vi "Read Scaled Async Data.vi"(8 "error in (no error)":errorcluster, 10 "Async Message":refnum<class "Async Message.lvclass">, 11 "1553 Component in":refnum<class "1553 Component.lvclass">) -> (0 "error out":errorcluster, 1 "Scaled Data":dbl[](array[numeric]), 2 "Parameters":string[](array[string]), 3 "1553 Component out":refnum<class "1553 Component.lvclass">)   [LabVIEW 2020, in "BCI-1553 API.lvlib" / "1553 Component.lvclass"]
doc: "Reads the parameters and values associated with an asynchronous message that was sent out on a Bus Controller. Data will be rescaled to engineering values depending on the configuration of the asynchronous message."
uses:
  1553 Component.lvclass
  Frames & Messages/Async Message/Async Message.lvclass
  1553 Component.lvclass/1553 Component.ctl
  Bus Controller/Bus Controller.lvclass
  C:/Users/MattJ/Desktop/git/bci-1553-labview-api/src/RealTime/1553 SubComponent/1553 SubComponent.lvclass
  1553 SubComponent/1553 SubComponent.lvclass
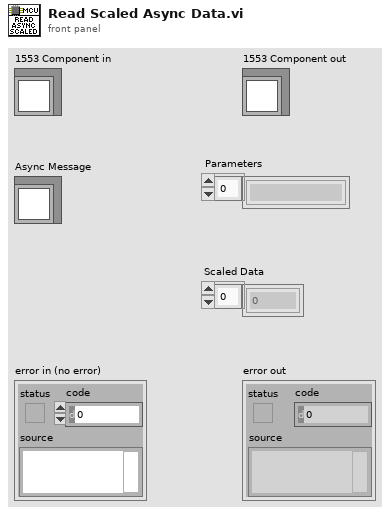
[diagram p1: front panel]
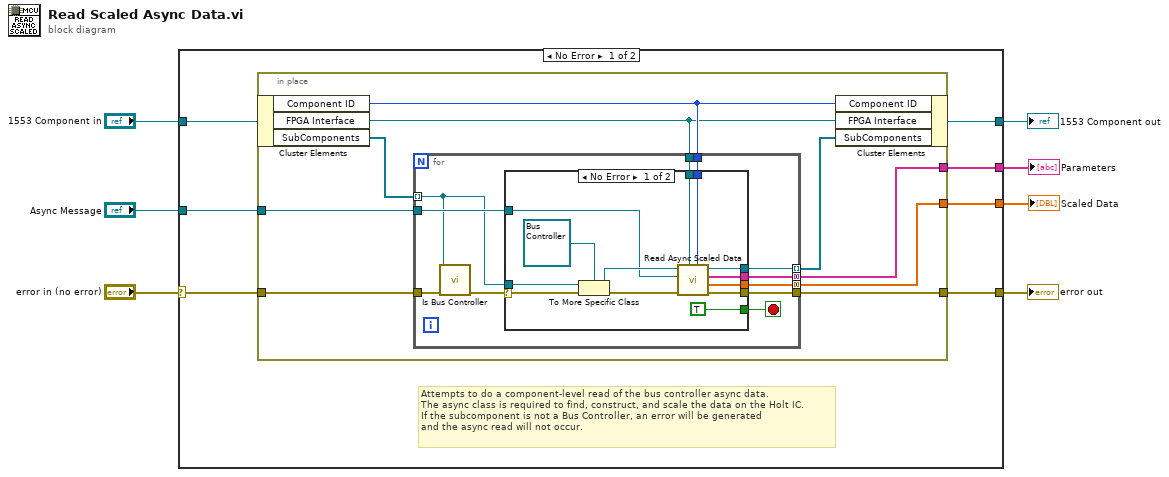
[diagram p0: block diagram]
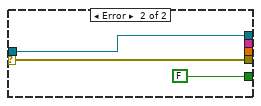
[diagram p2: hidden frame]
diagram:
  n1 = case shown="No Error" "error in (no error)" {
    selector: "error in (no error)" -> [w12 w52]
    tunnel: [w11 w52] -> w5
    tunnel: [w13 w51] -> w6
    tunnel: "1553 Component in" -> [w14 w51]
    tunnel: [w10 _] -> w2
    tunnel: [w9 _] -> w1
    tunnel: "Async Message" -> [w8 _]
    frame No Error {
      # "Attempts to do a component-level read of the bus controller async data.\nThe async class is required to find, construct, and scale the data on the Holt IC.\nIf the subcomponent is not a Bus Controller, an error will be generated\nand the async read will not occur."
      n2 = in-place {
        in-place-border: w12 -> [w19]
        in-place-border: [w18] -> w11
        in-place-border: [w17] -> w10
        in-place-border: [w16] -> w9
        in-place-border: w8 -> [w15]
        n3 = in-place-cluster #1(w14) -> ("Component ID"=w23:u8, "FPGA Interface"=w20:refnum<class "FPGA Interface.lvclass">, "SubComponents"=w22:refnum<class "1553 SubComponent.lvclass">[])
        n4 = for {
          tunnel: w22 -> [w24] mode=indexing
          tunnel: [w32] -> w21 mode=indexing
          tunnel: w23 -> [w34]
          tunnel: w20 -> [w33]
          tunnel: [w31] -> w17 mode=concatenating
          tunnel: [w30] -> w16 mode=concatenating
          tunnel: w15 -> [w25]
          tunnel: w19 -> [w28]
          tunnel: [w29] -> w18
          stop <- w26 stop-if-true
          n5 = call "Is Bus Controller.vi"("error in (no error)"=w28, "1553 SubComponent"=w24) -> ("error out"=w27:errorcluster)  [unwired: 9 in]
          n6 = case shown="No Error" w27 {
            selector: w27 -> [w45 w49]
            tunnel: w34 -> [w42 _]
            tunnel: w33 -> [w43 _]
            tunnel: [w41 w50] -> w32
            tunnel: [w36 _] -> w31
            tunnel: [w35 _] -> w30
            tunnel: [w37 w49] -> w29
            tunnel: w24 -> [w46 w50]
            tunnel: [TRUE FALSE] -> w26
            tunnel: w25 -> [w39 _]
            frame No Error {
              n7 = To More Specific Class(target class=refnum<class "Bus Controller.lvclass"> refnum ("SLSC 1553 API.lvlib:Bus Controller.lvclass"), reference=w46, error in=w45) -> (specific class reference=w40:refnum<class "Bus Controller.lvclass">, error out=w38:errorcluster)
              n8 = call-dynamic "Read Async Scaled Data.vi"("Component ID"=w42, "FPGA Interface"=w43, "error in (no error)"=w38, "Async Message"=w39, "Bus Controller in"=w40) -> ("error out"=w37:errorcluster, "Parameter Data"=w35:dbl[], "Parameters"=w36:string[], "Bus Controller out"=w41:refnum<class "Bus Controller.lvclass">)  [unwired: 3 in]
            }
            frame Error {
            }
          }
        }
        n9 = in-place-cluster #1("Component ID"=w23, "FPGA Interface"=w20, "SubComponents"=w21) -> (w13:refnum<class "1553 Component.lvclass">)
      }
    }
    frame Error {
    }
  }
  "error out" <- w5
  "1553 Component out" <- w6
  "Parameters" <- w2
  "Scaled Data" <- w1
